vi "characters.get.vi"(8 "error in (no error)":errorcluster, 11 "issue_class in":refnum<class "issue_class.lvclass">) -> (0 "error out":errorcluster, 1 "id":string, 2 "characters":T1[](array[typedef]), 3 "issue_class out":refnum<class "issue_class.lvclass">)   [LabVIEW 2024, in "issue_class.lvclass"]
uses:
  issue_class.lvclass
  definitions/character.ctl
  issue_class.lvclass/issue_class.ctl
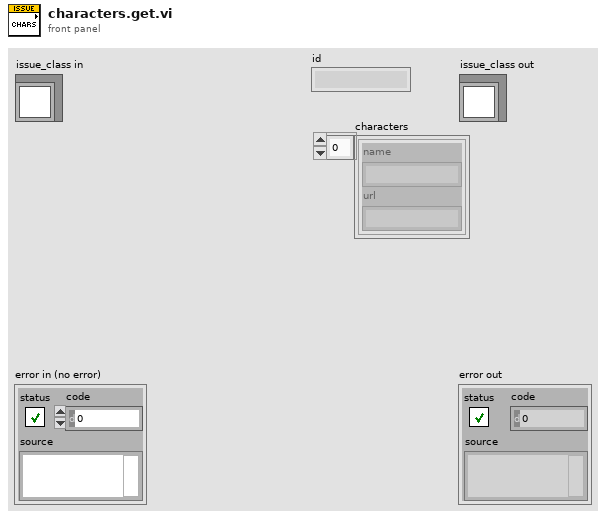
[diagram p1: front panel]
types:
  T1 = typedef "character.ctl" = cluster{"name":string, "url":string}
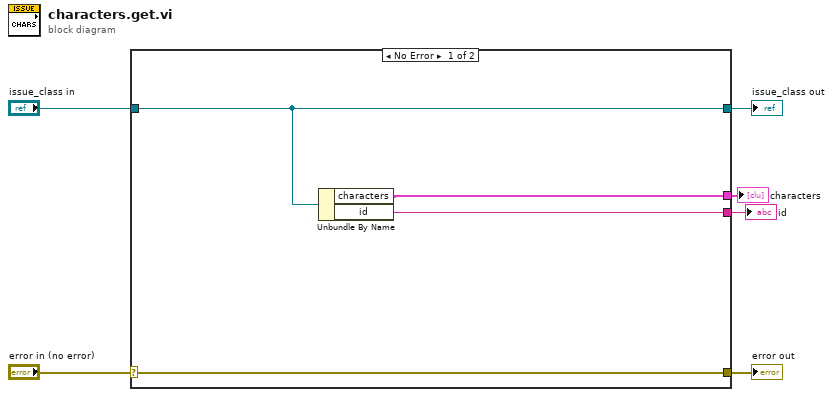
[diagram p0: block diagram]
diagram:
  n1 = case shown="No Error" "error in (no error)" {
    selector: "error in (no error)" -> [w10 w12]
    tunnel: [w10 w12] -> w5
    tunnel: [w9 w11] -> w3
    tunnel: "issue_class in" -> [w9 w11]
    tunnel: [w8 _] -> w2
    tunnel: [w7 _] -> w1
    frame No Error {
      n2 = Unbundle By Name(w9) -> ("characters"=w8:T1[], "id"=w7:string)
    }
    frame Error {
    }
  }
  "error out" <- w5
  "issue_class out" <- w3
  "characters" <- w2
  "id" <- w1
